vi "File-Close aborted files.vi"() -> ()   [LabVIEW 2020]
uses:
  Global Variables/General Globals.vi
panel:
  out "Array":errorcluster[](array[cluster])
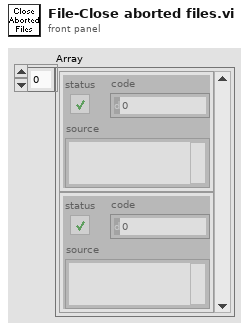
[diagram p1: front panel]
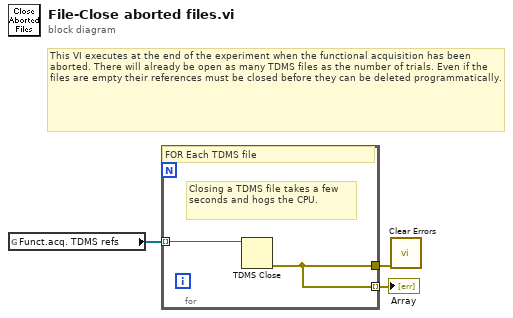
[diagram p0: block diagram]
diagram:
  # "This VI executes at the end of the experiment when the functional acquisition has been aborted. There will already be open as many TDMS files as the number of trials. Even if the files are empty their references must be closed before they can be deleted programmatically."
  n1 = global read "General Globals.vi" "Funct.acq. TDMS refs"() -> (w2:refnum<k34>[])
  n2 = for {
    tunnel: [w4] -> w3
    tunnel: w2 -> [w5] mode=indexing
    tunnel: [w4] -> w1 mode=indexing
    # "Closing a TDMS file takes a few seconds and hogs the CPU."
    # "FOR Each TDMS file"
    n3 = TDMS Close(11:w5) -> (0:w4:errorcluster)  [unwired: 1 in, 1 out]
  }
  "Array" <- w1
  n4 = call <vilib>:"Clear Errors.vi"("error in (no error)"=w3) -> ()  [unwired: 5 in, 2 out]
